vi "getRFChannel.vi"(8 "error in (no error)":errorcluster, 11 "rf.lvclass in":refnum<class "rf.lvclass">) -> (0 "error out":errorcluster, 2 "RfOutputChannel.lvclass":refnum<class "RfOutputChannel.lvclass">, 3 "rf.lvclass out":refnum<class "rf.lvclass">)   [LabVIEW 2009, in "Tools.lvlib" / "Scripting.lvlib" / "rf.lvclass"]
uses:
  rf.lvclass
  DatabaseHelpers/Database Objects/Channel/RfOutputChannel/RfOutputChannel.lvclass
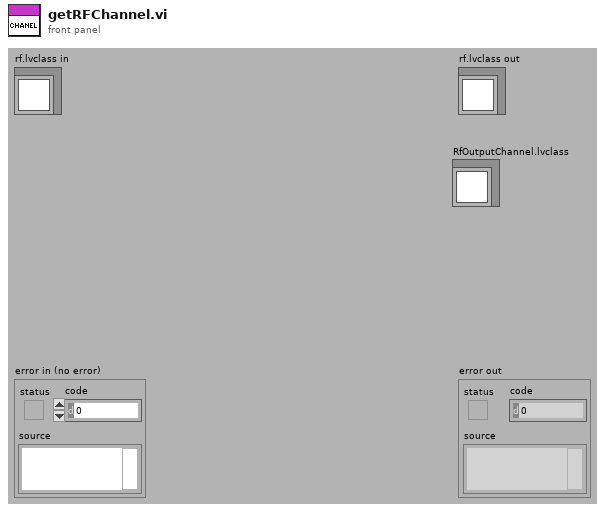
[diagram p1: front panel]
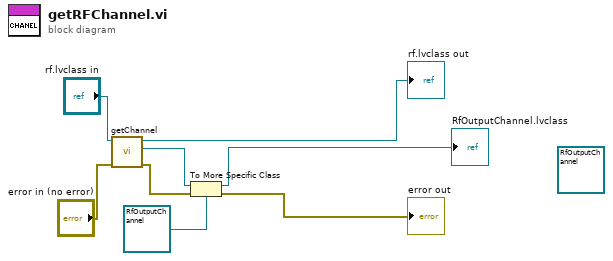
[diagram p0: block diagram]
diagram:
  (unwired) refnum<class "RfOutputChannel.lvclass"> refnum ("Tools.lvlib:DatabaseHelpers.lvlib:RfOutputChannel.lvclass")
  n1 = call-dynamic "getChannel.vi"("error in (no error)"="error in (no error)", "ScriptEvent.lvclass in"="rf.lvclass in") -> ("error out"=w1:errorcluster, "Channel.lvclass"=w4:refnum<class "Channel.lvclass">, "ScriptEvent.lvclass out"=→"rf.lvclass out":refnum<class "rf.lvclass">)  [unwired: 7 in]
  n2 = To More Specific Class(target class=refnum<class "RfOutputChannel.lvclass"> refnum ("Tools.lvlib:DatabaseHelpers.lvlib:RfOutputChannel.lvclass"), reference=w4, error in=w1) -> (specific class reference=→"RfOutputChannel.lvclass":refnum<class "RfOutputChannel.lvclass">, error out=→"error out":errorcluster)
